vi "SVPO Scale Voltage to EU (1 Ch SGL WDT).vi"(7 "write waveform attributes? (T)":bool=TRUE, 10 "channel info":T1={"sensor sensitivity"=1000.0, "engineering units"=1, "dB reference"=1.0, "custom label"="EU", "weighting filter"=0, "pregain"=0.0} {"pregain" format="%.2f"; "weighting filter" items=["Linear", "A-weighting", "B-weighting", "C-weighting", "ITU-R 468-4", "Dolby", "CCITT", "C-message", "Wb", "Wc", "Wd", "We", "Wf", "Wh", "Wj", "Wk", "Wm", "AES17 20 kHz lowpass", "AES17 40 kHz lowpass", "AES17 20 kHz highpass", "AES17 40 kHz highpass"]; "dB reference" format="%^.1e"; "engineering units" items=["custom..."=0, "V"=1, "A"=21, "C"=30, "pC"=31, "s"=32, "-"=29, "Pa"=2, "N"=20, "g"=3, "m/s^2"=4, "m/s"=5, "m"=6, "mm/s"=12, "mm"=13, "micron/s"=14, "micron"=15, "in/s^2"=7, "in/s"=8, "in"=9, "mil/s"=10, "mil"=11, "rad/s^2"=16, "rad/s"=17, "rad"=18, "deg/s^2"=26, "deg/s"=27, "deg"=28, "RPM"=22, "cycle/s^2"=23, "Hz"=24, "cycle"=25, "strain"=19]; "sensor sensitivity" format="%#_5f"}, 11 "signal [V]":waveform(sgl)={"t0"=timestamp(0 s since 1904-01-01), "dt"=0.0, "Y"=[]}) -> (3 "scaled signal [EU]":waveform(sgl))   [LabVIEW 2017, in "SoundVib_Calibration.lvlib"]
doc: "Scales the single-precision <B>signal [V]</B> from volts to the engineering units (EU) you select. Scale signals to appropriate EU before applying limits, saving to disk, and performing measurement analyses. Use this VI on embedded targets that have limited computational resources. Wire data to the <B>signal [V]</B> input to determine the polymorphic instance to use or manually select the instance."
uses:
  <vilib>/addons/Sound and Vibration/svt_Calibration/SoundVib_Calibration.lvlib
  <vilib>/addons/_NISVFA/_Shared subVIs/Controls/svc_Channel Info.ctl
  <vilib>/addons/_NISVFA/_Shared subVIs/Controls/svc_Engineering Units Text Ring.ctl
  <vilib>/addons/_NISVFA/_Shared subVIs/Controls/svc_Weighting Filter Text Ring.ctl
  <vilib>/addons/_NISVFA/_Shared subVIs/Common/svc_Set SV Channel Info (variant).vi
  <vilib>/addons/_NISVFA/_Shared subVIs/Common/SVL Set dB Reference (variant).vi
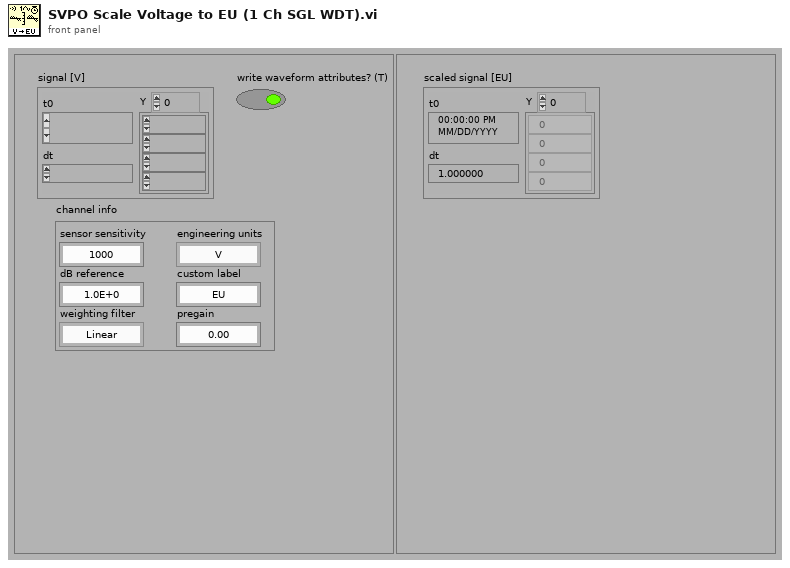
[diagram p1: front panel]
types:
  T1 = typedef "svc_Channel Info.ctl" = cluster{"sensor sensitivity":dbl, "engineering units":T2, "dB reference":dbl, "custom label":string, "weighting filter":T3, "pregain":dbl}
  T2 = typedef "svc_Engineering Units Text Ring.ctl" = u16
  T3 = typedef "svc_Weighting Filter Text Ring.ctl" = u16
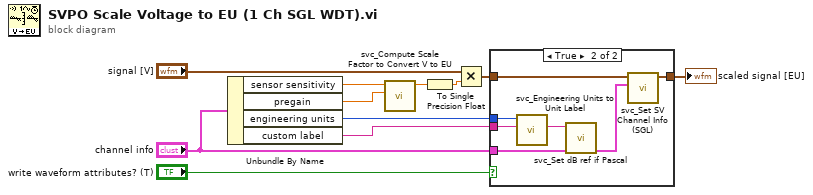
[diagram p0: block diagram]
diagram:
  n1 = Unbundle By Name("channel info") -> ("sensor sensitivity"=w5:dbl, "pregain"=w6:dbl, "engineering units"=w1:T2, "custom label"=w2:string)
  n2 = call <vilib>:"svc_Compute Scale Factor to Convert V to EU.vi"("pregain [dB]"=w6, "sensor sensitivity [mV/EU]"=w5) -> ("EU scale factor [EU/V]"=w3:dbl)  [unwired: 9 in]
  n3 = To Single Precision Float(number=w3) -> (single precision float=w8:sgl)
  n4 = Multiply(x="signal [V]", y=w8) -> (x*y=w10:waveform(sgl))
  n5 = case shown="True" "write waveform attributes? (T)" {
    tunnel: "channel info" -> [_ w19]
    tunnel: w10 -> [w12 w18]
    tunnel: [w12 w17] -> w9
    tunnel: w2 -> [_ w15]
    tunnel: w1 -> [_ w14]
    frame False {
    }
    frame True {
      n6 = call <vilib>:"svc_Engineering Units to Unit Label.vi"("custom label"=w15, "engineering units"=w14) -> ("unit label"=w13:string)  [unwired: 8 in, 1 out]
      n7 = call <vilib>:"svc_Set dB ref if Pascal.vi"("channel info"=w19, "unit label"=w13) -> ("channel info"=w16:T1)  [unwired: 4 in, 1 out]
      n8 = call <vilib>:"svc_Set SV Channel Info (SGL).vi"("channel info"=w16, "scaled signal in"=w18) -> ("scaled signal out"=w17:waveform(sgl))  [unwired: 8 in, 1 out]
    }
  }
  "scaled signal [EU]" <- w9
